vi "Get Instrument VIs.vi"(8 "error in":errorcluster, 10 "instr containing vis":path[](array[path]), 11 "destination directory":path) -> (0 "error out":errorcluster, 3 "new paths of instr containing vis":path[](array[path]))   [LabVIEW 2021, in "Converter.lvlib"]
uses:
  Converter.lvlib
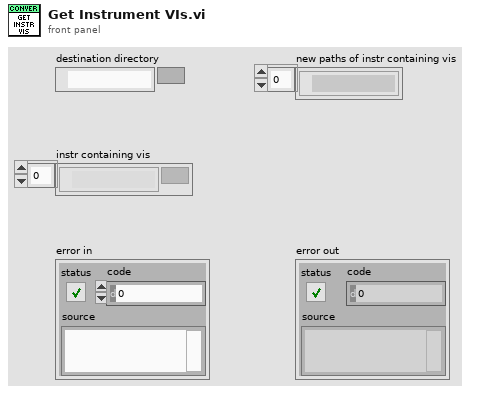
[diagram p1: front panel]
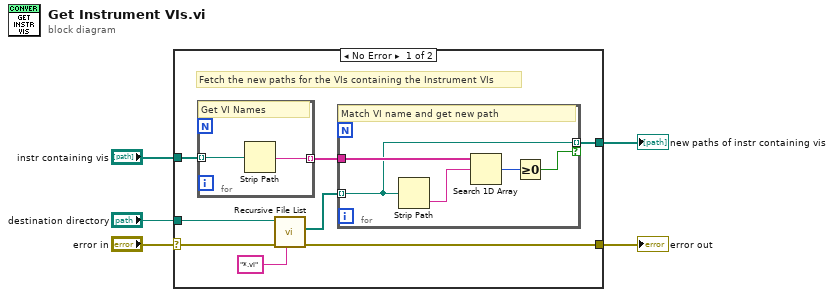
[diagram p0: block diagram]
diagram:
  n1 = case shown="No Error" "error in" {
    selector: "error in" -> [w8 w21]
    tunnel: [w13 w21] -> w5
    tunnel: [w12 _] -> w4
    tunnel: "instr containing vis" -> [w11 _]
    tunnel: "destination directory" -> [w7 _]
    frame No Error {
      # "Fetch the new paths for the VIs containing the Instrument VIs"
      n2 = for {
        tunnel: w11 -> [w20] mode=indexing
        tunnel: [w19] -> w10 mode=indexing
        # "Get VI Names"
        n3 = Strip Path(path=w20) -> (name=w19:string)  [unwired: 1 out]
      }
      n4 = call <vilib>:"Recursive File List.vi"("pattern"="*.vi", "error in (no error)"=w8, "Folder Path"=w7) -> ("error out"=w13:errorcluster, "All Files in Dir"=w9:path[])  [unwired: 4 in, 3 out]
      n5 = for {
        tunnel: w9 -> [w15] mode=indexing
        tunnel: w10 -> [w18]
        tunnel: [w15] -> w12 mode=indexing if=w14
        # "Match VI name and get new path"
        n6 = Strip Path(path=w15) -> (name=w17:string)  [unwired: 1 out]
        n7 = Search 1D Array(1D array=w18, element=w17) -> (index of element=w16:i32)  [unwired: 1 in]
        n8 = Greater Or Equal To 0?(x=w16) -> (x >= 0?=w14:bool)
      }
    }
    frame Error {
    }
  }
  "error out" <- w5
  "new paths of instr containing vis" <- w4
